vi "Arayuz_v4.vi"() -> ()   [LabVIEW 2014]
uses:
  CustomControls/Program_States.ctl
  <vilib>/Platform/TimedLoop/XDataNode/timing_clust.ctl
  <vilib>/Platform/TimedLoop/XDataNode/nitl_modes.ctl
  <vilib>/Platform/TimedLoop/XDataNode/wakeup.ctl
  CustomControls/TSE_Status.ctl
  SharedVariables/TSE_Variables.vi
  <vilib>/platform/TimedLoop/XDataNode/XDataNode.xnode
  <vilib>/Platform/TimedLoop/XDataNode/XDNodeRunTimeDep.lvlib
panel:
  in  "?":string="GKÇ KALİBRASYON YAZILIMI"
  in  "Sertifika Kaydet":bool=TRUE
  in  "DURDUR":bool
  out "Ring":T1=enum."Durdur"
  in  "Main Tab Control":enum32{"GKÇ 1", "GKÇ 2", "GKÇ 3"}(tab)
  in  "GKÇ-1 Tab Control":T2(tab)
  out "GKÇ-1 Frekans Sonuç Tablosu":string[][](table)
  out "GKÇ-1 Gerilim Sonuç Tablosu":string[][](table)
  out "GKÇ-1 Akım Sonuç Tablosu":string[][](table)
  out "GKÇ-1 Aktif Güç Sonuç Tablosu":string[][](table)
  out "GKÇ-1 Reaktif Güç Sonuç Tablosu":string[][](table)
  out "GKÇ-1 Harmonik Akım Sonuç Tablosu":string[][](table)
  out "GKÇ-1 Harmonik Gerilim Sonuç Tablosu":string[][](table)
  out "GKÇ-1 Flicker Sonuç Tablosu":string[][](table)
  out "Flicker Sonuç":bool caption="Flicker"
  out "Harmonik G. Sonuç":bool caption="Harmonik Gerilim"
  out "Harmonik A. Sonuç":bool caption="Harmonik Akım"
  out "Reaktif G. Sonuç":bool caption="Reaktif Güç"
  out "Aktif G. Sonuç":bool caption="Aktif Güç"
  out "Akım Sonuç":bool caption="AC Akım"
  out "Gerilim Sonuç":bool caption="AC Gerilim"
  out "Mesaj":string="Program Durduruldu !"
  out "Frekans Sonuç":bool caption="Frekans"
  in  "Dosya Adı":path
  in  "BAŞLAT":bool
  # "Uygulanan Değer"
  # "Hata_Fider 1"
  # "Hata_Fider 2"
  # "Sonuç"
  # "Uygulanan Değer"
  # "Hata_Fider 1"
  # "Hata_Fider 2"
  # "Sonuç"
  # "Uygulanan Değer"
  # "Hata_Fider 1"
  # "Hata_Fider 2"
  # "Sonuç"
  # "Uygulanan Değer"
  # "Hata_Fider 1"
  # "Hata_Fider 2"
  # "Sonuç"
  # "Uygulanan Değer"
  # "Hata_Fider 1"
  # "Hata_Fider 2"
  # "Sonuç"
  # "Uygulanan Değer"
  # "Hata_Fider 1"
  # "Hata_Fider 2"
  # "Sonuç"
  # "Uygulanan Değer"
  # "Hata_Fider 1"
  # "Hata_Fider 2"
  # "Sonuç"
  # "Uygulanan Değer"
  # "Hata_Fider 1"
  # "Hata_Fider 2"
  # "Sonuç"
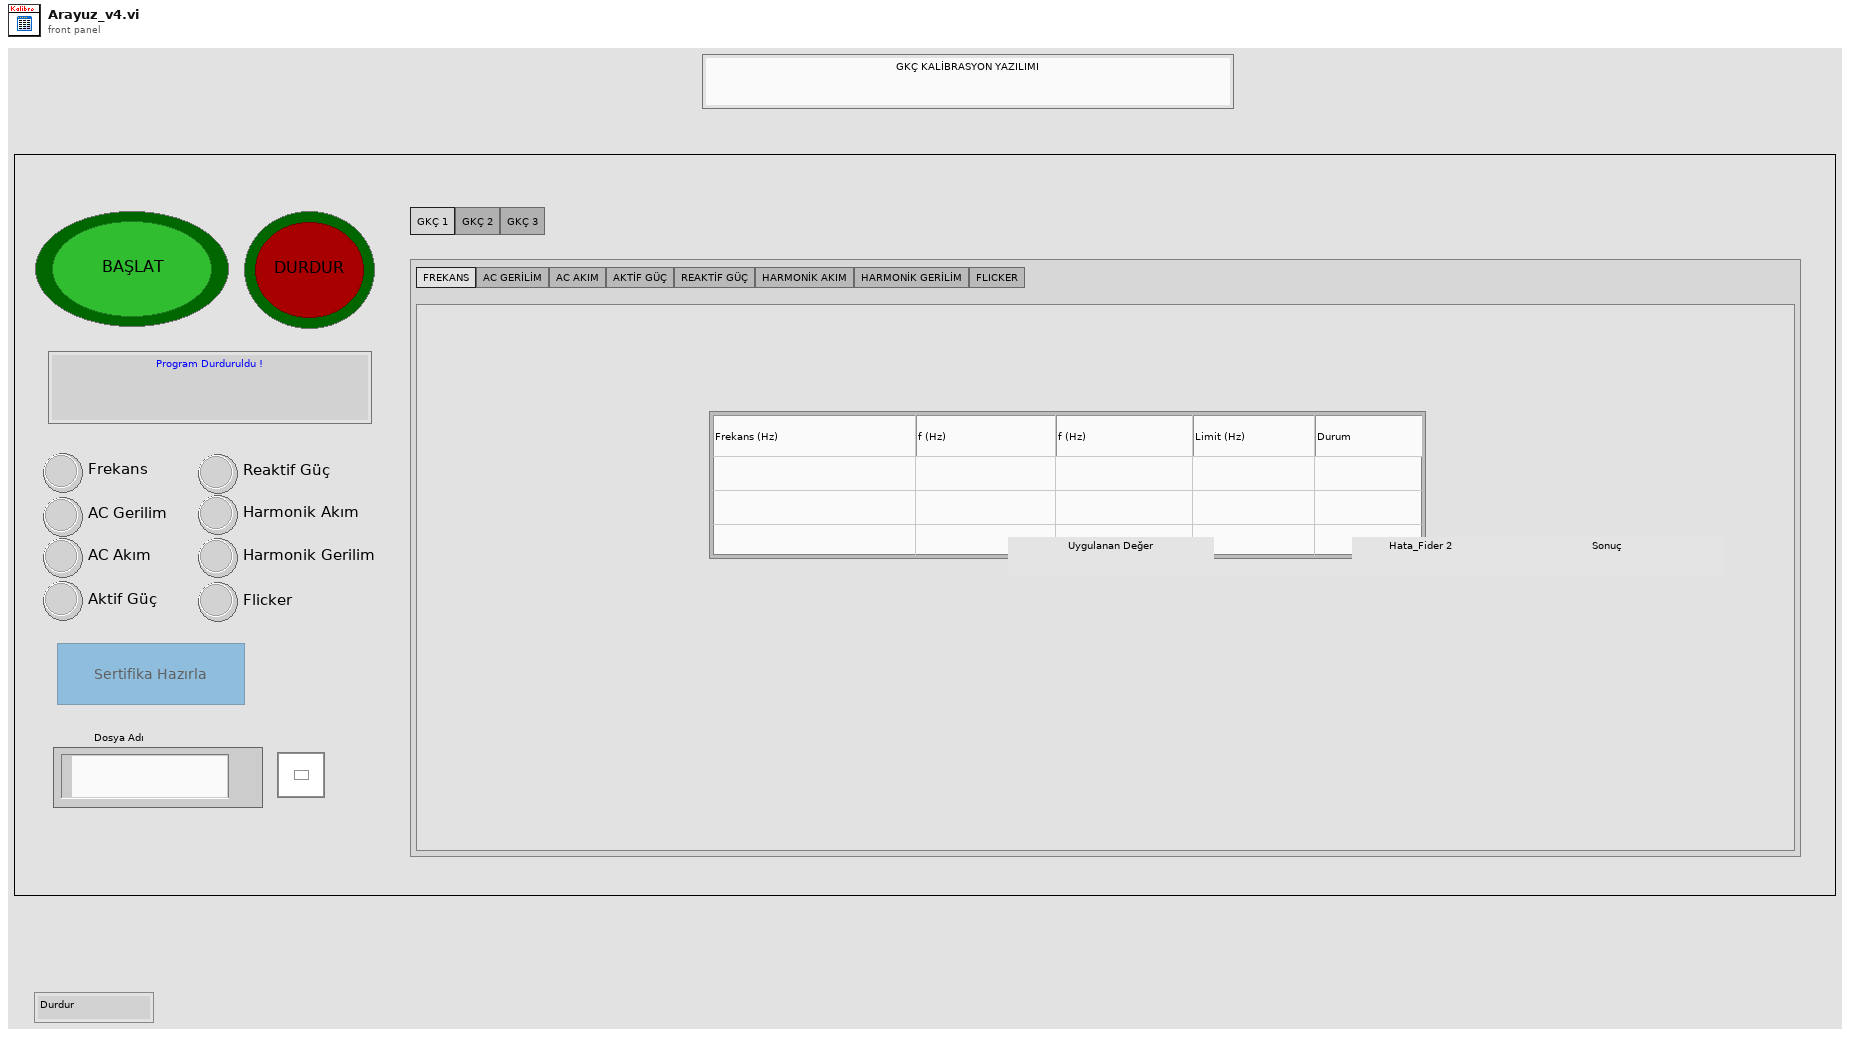
[diagram p1: front panel]
types:
  T1 = typedef "Program_States.ctl" = enum16{"Ön Yükleme", "TSE Baslat", "Kalibratöre Baglan", "Kalibratörü Baslat", "Ön Yükleme Tamam", "Frekans Testi", "Gerilim Testi", "Akim Testi", "Aktif Guc Testi", "Reaktif Guc Testi", "AC Akim Harmonik Testi", "AC Gerilim Harmonik Testi", "Flicker Testi", "Rapor Cikarma", "Yeniden Başlat", "Bekleme", "Durdur"}
  T2 = enum32{"FREKANS", "AC GERİLİM", "AC AKIM", "AKTİF GÜÇ", "REAKTİF GÜÇ", "HARMONİK AKIM", "HARMONİK GERİLİM", "FLICKER"}
  T3 = cluster{"Test A. Süresi":i32, "Iterasyon Sayisi":i32}
  T4 = typedef "TSE_Status.ctl" = cluster{"Return Code":i32, "Message":string, "error in (no error)":errorcluster, "Program State":T1, "Test A. Suresi":u32}
  T5 = typedef "XDNodeRunTimeDep.lvlib/timing_clust.ctl" = cluster{"Expected End [f-1]":u64, "Actual End [f-1]":u64, "Finished Late? [f-1]":bool, "Expected End [i-1]":u64, "Actual End [i-1]":u64, "Finished Late? [i-1]":bool, "Expected Start [i]":u64, "Actual Start [i]":u64, "Expected Start [f]":u64, "Actual Start [f]":u64, "Source Name":string, "Structure Name":string, "Period":i64, "Deadline":i64, "Offset":i64, "Start":i64, "Priority":i32, "Timeout":i32, "Mode":T6, "Wakeup Reason":T7, "Error":errorcluster, "Source Type":string, "Secondary Source Type":string, "Global End Time":u64, "Global Start Time":u64, "Frame Duration":u64, "Iteration Duration":u64, "Assigned CPU":i32, "I/O Scan Engine Mode":u32}
  T6 = typedef "XDNodeRunTimeDep.lvlib/nitl_modes.ctl" = enum32{"No Change", "Process missed periods, maintain original phase", "Discard missed periods, maintain original phase", "Process missed periods, ignore original phase", "Discard missed periods, ignore original phase"}
  T7 = typedef "XDNodeRunTimeDep.lvlib/wakeup.ctl" = enum32{"Normal", "Aborted", "Asynchronous wakeup", "Timing source error", "Timed loop error", "Timeout"}
  T8 = enum8{"Enabled", "Disabled", "Disabled and Grayed Out"}
  T9 = enum32{"invalid app kind", "Development System", "Run Time System", "Student Edition", "Embedded LabVIEW", "Evaluation", "Custom"}
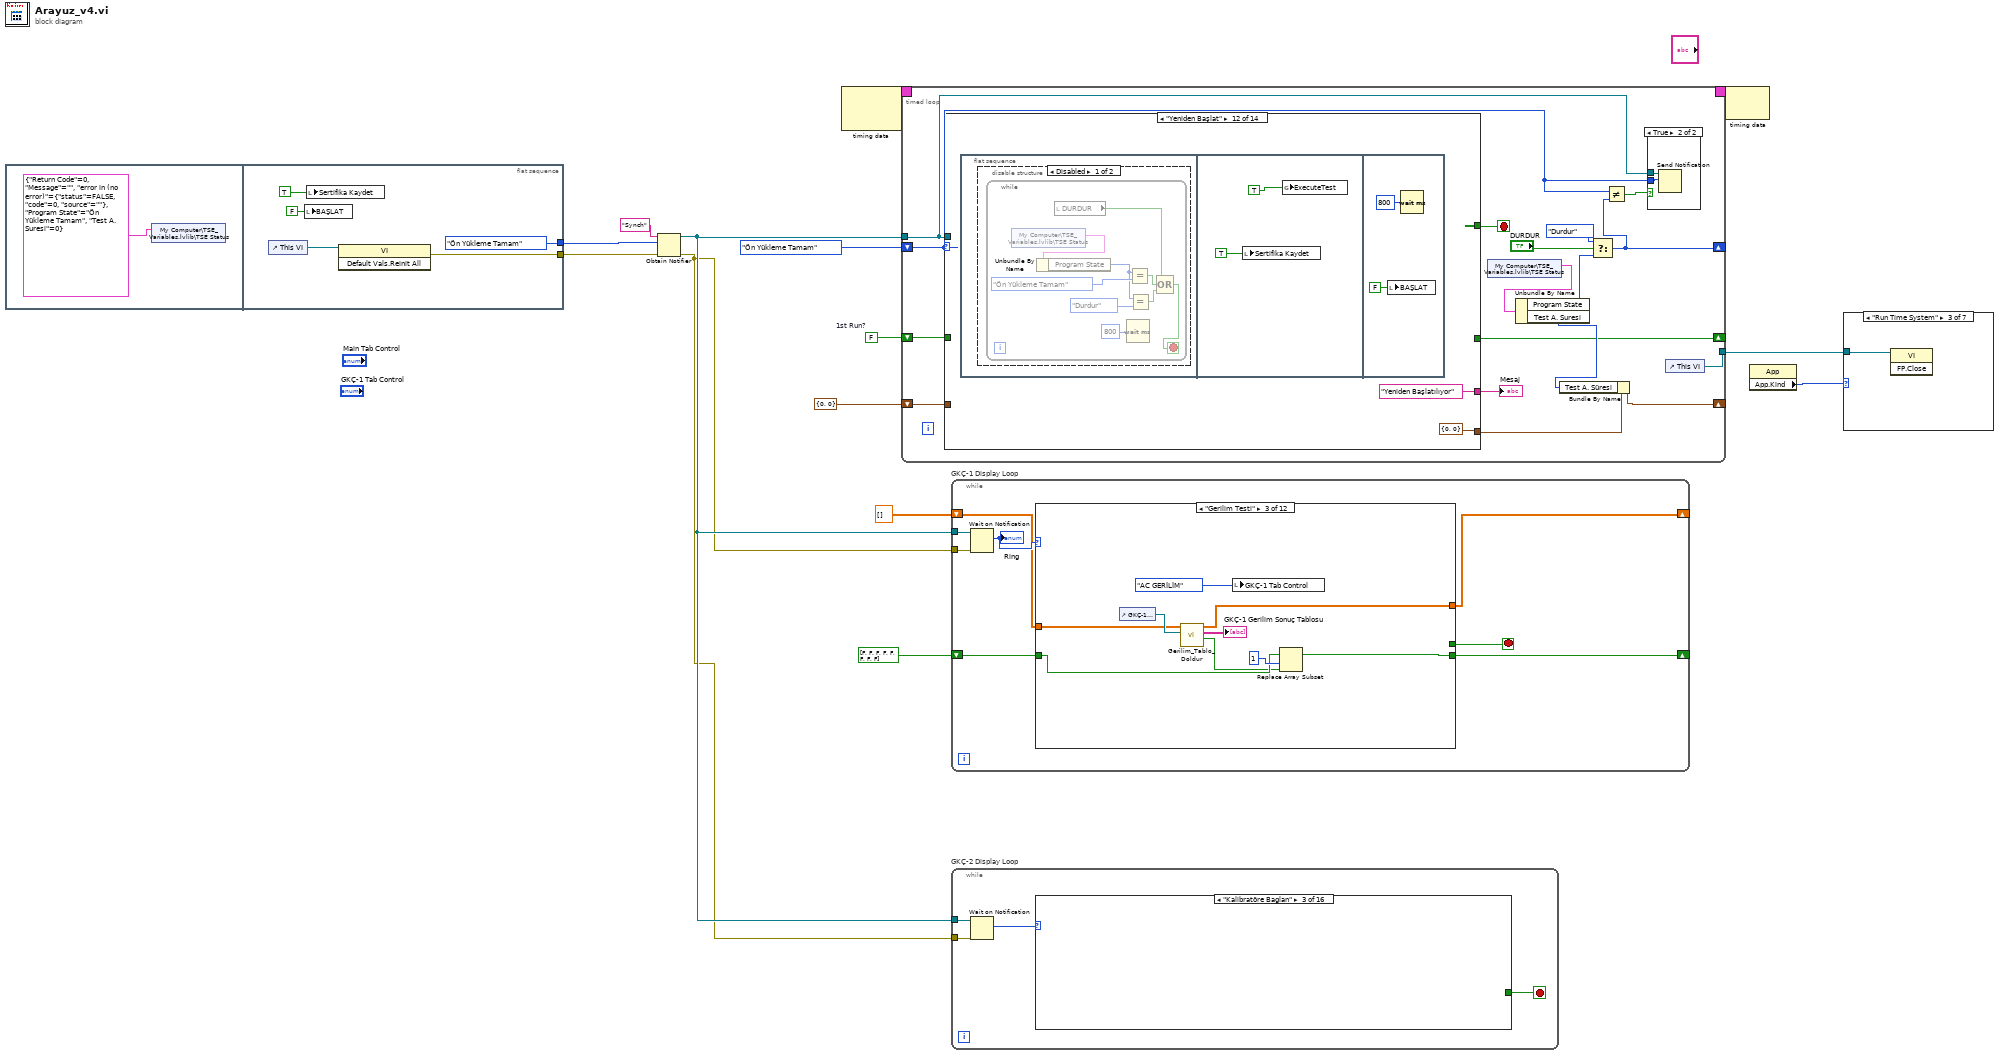
[diagram p0: block diagram]
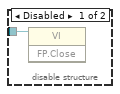
[diagram p4: hidden frame]
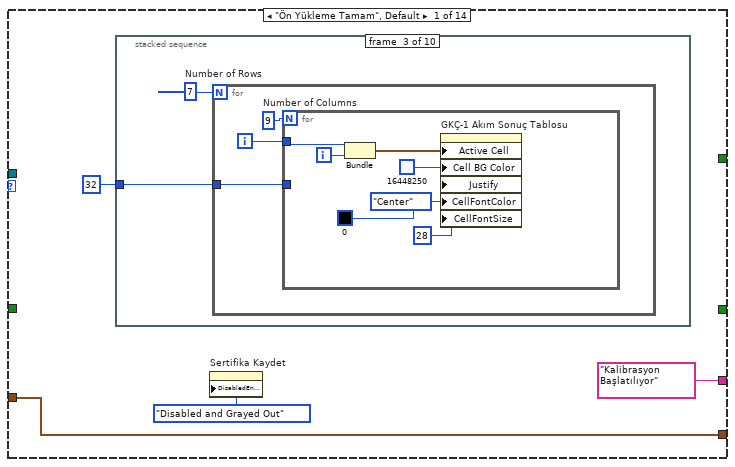
[diagram p10: hidden frame]
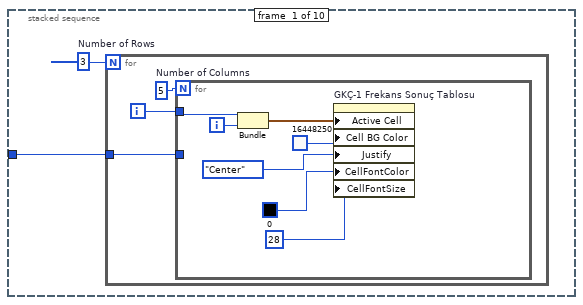
[diagram p11: hidden frame]
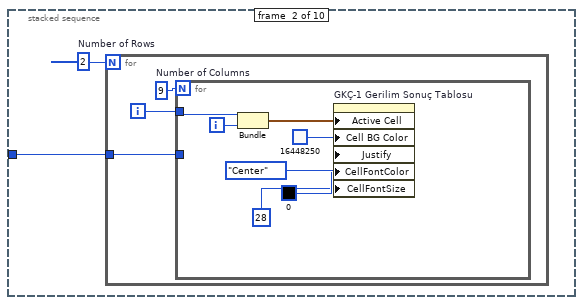
[diagram p12: hidden frame]
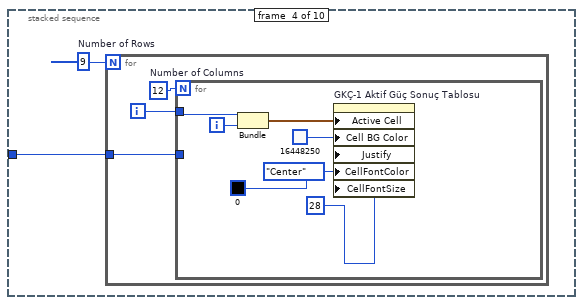
[diagram p13: hidden frame]
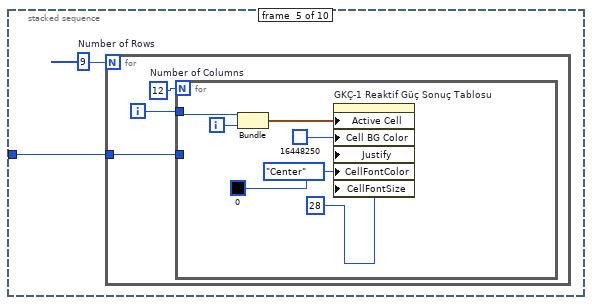
[diagram p14: hidden frame]
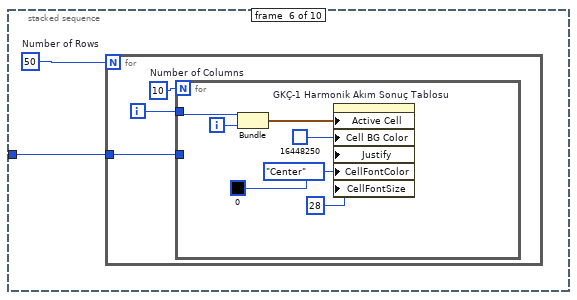
[diagram p15: hidden frame]
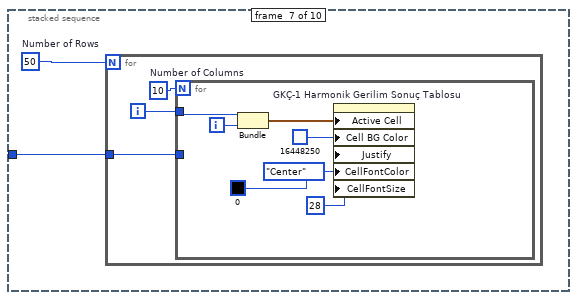
[diagram p16: hidden frame]
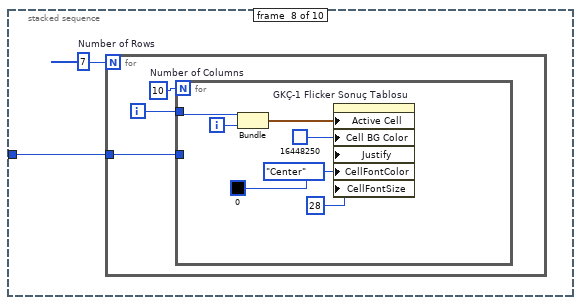
[diagram p17: hidden frame]
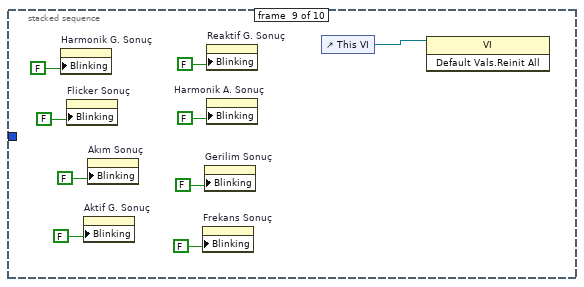
[diagram p18: hidden frame]
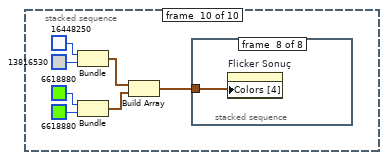
[diagram p19: hidden frame]
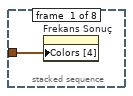
[diagram p20: hidden frame]
diagram:
  w2 = FALSE  # 1st Run?
  n1 = flat-sequence {
    tunnel: [Program_States."Ön Yükleme Tamam" ("Ring")] -> w13
    tunnel: [w18] -> w6
    frame #0 {
      n2 = shared-variable "My Computer\\TSE_Variables.lvlib\\TSE Status"(T4 {"Return Code"=0, "Message"="", "error in (no error)"={"status"=FALSE, "code"=0, "source"=""}, "Program State"=enum."Ön Yükleme Tamam", "Test A. Suresi"=0} ("TSE Status")) -> ()  [unwired: 1 in, 1 out]
    }
    frame #1 {
      n3 = control-ref of="This VI"() -> (w19:refnum<vi>)
      n4 = local write "BAŞLAT"(FALSE ("BAŞLAT")) -> ()
      n5 = local write "Sertifika Kaydet"(TRUE ("Sertifika Kaydet")) -> ()
      n6 = invoke class="VI" method="Default Vals.Reinit All"(reference=w19) -> (error out=w18:errorcluster)  [unwired: 2 in, 2 out]
    }
  }
  n7 = Obtain Notifier(name (unnamed)="Synch", notification data type=w13, error in (no error)=w6) -> (notifier out=w11:refnum<notifier>, error out=w10:errorcluster)  [unwired: 1 in, 1 out]
  n8 = node-c288() -> (w8:T5)  [unwired: 2 in]
  n9 = timed-loop {
    tunnel: w11 -> [w26]
    shift-right: [w27] -> _
    shift-left: Program_States."Ön Yükleme Tamam" ("Ring") -> [w24]
    shift-right: [w33] -> _
    shift-left: T3 {"Test A. Süresi"=0, "Iterasyon Sayisi"=0} -> [w37]
    timing: w8 -> [_]
    timing-out: [_] -> w7
    tunnel: [w28] -> w5
    shift-right: [w22] -> _
    shift-left: w2 -> [w23]
    stop <- w31 stop-if-true
    n10 = case shown="\"Yeniden Başlat\"" w24 {
      selector: w24 -> [_ _ _ _ _ _ _ _ _ _ _ _ w315 w326]
      tunnel: w37 -> [w43 _ w173 w184 w199 w214 w230 w243 w258 w273 _ _ _ w329]
      tunnel: [w43 _ w170 w181 w196 w211 w227 w240 w255 w270 _ T3 {"Test A. Süresi"=0, "Iterasyon Sayisi"=0} _ w328] -> w36
      tunnel: [_ _ FALSE FALSE FALSE FALSE FALSE FALSE FALSE FALSE _ _ TRUE _] -> w31
      tunnel: ["Kalibrasyon Başlatılıyor" "" "Frekans Ölçümü\nDevam Ediyor" w186 w201 w216 "Reaktif Güç Ölçümü\nDevam Ediyor" w245 w260 w275 "Ölçümler Tamamlandı" "Yeniden Başlatılıyor" "Program Durduruldu !" "Bekleniyor..."] -> w30
      tunnel: w26 -> [_ _ _ _ _ _ _ _ _ _ w285 _ w316 w325]
      tunnel: w23 -> [_ _ w167 w179 w194 w209 w224 w238 w253 w268 _ _ _ _]
      tunnel: [_ TRUE _ w178 w193 w208 w223 w237 w252 w267 _ _ _ _] -> w22
      frame "Ön Yükleme Tamam", Default {
        n11 = stacked-sequence {
          tunnel: u32 32 ("Active Cell:Cell Size:Height") -> [w44 w56 w68 w80 w92 w104 w116 w128 _ _]
          frame #0 {
            w45 = 3  # Number of Rows
            n12 = for {
              N: w45 -> [_]
              tunnel: w44 -> [w47]
              i -> [w48]
              w46 = 5  # Number of Columns
              n13 = for {
                N: w46 -> [_]
                tunnel: w48 -> [w55]
                tunnel: w47 -> [_]
                i -> [w52]
                n14 = Bundle(w55, w52) -> (w54:cluster{i32, i32})  [unwired: 1 in]
                n15 = property on="GKÇ-1 Frekans Sonuç Tablosu" class="Tbl (strict)"("Active Cell"=w54, "Cell BG Color"=u32 16448250, "Justify"=enum16{"Left", "Center", "Right"}."Center" ("Active Cell:Cell Justification"), "CellFontColor"=u32 0, "CellFontSize"=u32 28 ("Active Cell:Cell Font:Size")) -> ()  [unwired: 2 in, 2 out]
              }
            }
          }
          frame #1 {
            w57 = 2  # Number of Rows
            n16 = for {
              N: w57 -> [_]
              tunnel: w56 -> [w59]
              i -> [w60]
              w58 = 9  # Number of Columns
              n17 = for {
                N: w58 -> [_]
                tunnel: w60 -> [w67]
                tunnel: w59 -> [_]
                i -> [w64]
                n18 = Bundle(w67, w64) -> (w66:cluster{i32, i32})  [unwired: 1 in]
                n19 = property on="GKÇ-1 Gerilim Sonuç Tablosu" class="Tbl (strict)"("Active Cell"=w66, "Cell BG Color"=u32 16448250, "Justify"=enum16{"Left", "Center", "Right"}."Center" ("Active Cell:Cell Justification"), "CellFontColor"=u32 0, "CellFontSize"=u32 28 ("Active Cell:Cell Font:Size")) -> ()  [unwired: 2 in, 2 out]
              }
            }
          }
          frame #2 {
            w69 = 7  # Number of Rows
            n20 = for {
              N: w69 -> [_]
              tunnel: w68 -> [w71]
              i -> [w72]
              w70 = 9  # Number of Columns
              n21 = for {
                N: w70 -> [_]
                tunnel: w72 -> [w79]
                tunnel: w71 -> [_]
                i -> [w76]
                n22 = Bundle(w79, w76) -> (w78:cluster{i32, i32})  [unwired: 1 in]
                n23 = property on="GKÇ-1 Akım Sonuç Tablosu" class="Tbl (strict)"("Active Cell"=w78, "Cell BG Color"=u32 16448250, "Justify"=enum16{"Left", "Center", "Right"}."Center" ("Active Cell:Cell Justification"), "CellFontColor"=u32 0, "CellFontSize"=u32 28 ("Active Cell:Cell Font:Size")) -> ()  [unwired: 2 in, 2 out]
              }
            }
          }
          frame #3 {
            w81 = 9  # Number of Rows
            n24 = for {
              N: w81 -> [_]
              tunnel: w80 -> [w83]
              i -> [w84]
              w82 = 12  # Number of Columns
              n25 = for {
                N: w82 -> [_]
                tunnel: w84 -> [w91]
                tunnel: w83 -> [_]
                i -> [w88]
                n26 = Bundle(w91, w88) -> (w90:cluster{i32, i32})  [unwired: 1 in]
                n27 = property on="GKÇ-1 Aktif Güç Sonuç Tablosu" class="Tbl (strict)"("Active Cell"=w90, "Cell BG Color"=u32 16448250, "Justify"=enum16{"Left", "Center", "Right"}."Center" ("Active Cell:Cell Justification"), "CellFontColor"=u32 0, "CellFontSize"=u32 28 ("Active Cell:Cell Font:Size")) -> ()  [unwired: 2 in, 2 out]
              }
            }
          }
          frame #4 {
            w93 = 9  # Number of Rows
            n28 = for {
              N: w93 -> [_]
              tunnel: w92 -> [w95]
              i -> [w96]
              w94 = 12  # Number of Columns
              n29 = for {
                N: w94 -> [_]
                tunnel: w96 -> [w103]
                tunnel: w95 -> [_]
                i -> [w100]
                n30 = Bundle(w103, w100) -> (w102:cluster{i32, i32})  [unwired: 1 in]
                n31 = property on="GKÇ-1 Reaktif Güç Sonuç Tablosu" class="Tbl (strict)"("Active Cell"=w102, "Cell BG Color"=u32 16448250, "Justify"=enum16{"Left", "Center", "Right"}."Center" ("Active Cell:Cell Justification"), "CellFontColor"=u32 0, "CellFontSize"=u32 28 ("Active Cell:Cell Font:Size")) -> ()  [unwired: 2 in, 2 out]
              }
            }
          }
          frame #5 {
            w105 = 50  # Number of Rows
            n32 = for {
              N: w105 -> [_]
              tunnel: w104 -> [w107]
              i -> [w108]
              w106 = 10  # Number of Columns
              n33 = for {
                N: w106 -> [_]
                tunnel: w108 -> [w115]
                tunnel: w107 -> [_]
                i -> [w112]
                n34 = Bundle(w115, w112) -> (w114:cluster{i32, i32})  [unwired: 1 in]
                n35 = property on="GKÇ-1 Harmonik Akım Sonuç Tablosu" class="Tbl (strict)"("Active Cell"=w114, "Cell BG Color"=u32 16448250, "Justify"=enum16{"Left", "Center", "Right"}."Center" ("Active Cell:Cell Justification"), "CellFontColor"=u32 0, "CellFontSize"=u32 28 ("Active Cell:Cell Font:Size")) -> ()  [unwired: 2 in, 2 out]
              }
            }
          }
          frame #6 {
            w117 = 50  # Number of Rows
            n36 = for {
              N: w117 -> [_]
              tunnel: w116 -> [w119]
              i -> [w120]
              w118 = 10  # Number of Columns
              n37 = for {
                N: w118 -> [_]
                tunnel: w120 -> [w127]
                tunnel: w119 -> [_]
                i -> [w124]
                n38 = Bundle(w127, w124) -> (w126:cluster{i32, i32})  [unwired: 1 in]
                n39 = property on="GKÇ-1 Harmonik Gerilim Sonuç Tablosu" class="Tbl (strict)"("Active Cell"=w126, "Cell BG Color"=u32 16448250, "Justify"=enum16{"Left", "Center", "Right"}."Center" ("Active Cell:Cell Justification"), "CellFontColor"=u32 0, "CellFontSize"=u32 28 ("Active Cell:Cell Font:Size")) -> ()  [unwired: 2 in, 2 out]
              }
            }
          }
          frame #7 {
            w129 = 7  # Number of Rows
            n40 = for {
              N: w129 -> [_]
              tunnel: w128 -> [w131]
              i -> [w132]
              w130 = 10  # Number of Columns
              n41 = for {
                N: w130 -> [_]
                tunnel: w132 -> [w139]
                tunnel: w131 -> [_]
                i -> [w136]
                n42 = Bundle(w139, w136) -> (w138:cluster{i32, i32})  [unwired: 1 in]
                n43 = property on="GKÇ-1 Flicker Sonuç Tablosu" class="Tbl (strict)"("Active Cell"=w138, "Cell BG Color"=u32 16448250, "Justify"=enum16{"Left", "Center", "Right"}."Center" ("Active Cell:Cell Justification"), "CellFontColor"=u32 0, "CellFontSize"=u32 28 ("Active Cell:Cell Font:Size")) -> ()  [unwired: 2 in, 2 out]
              }
            }
          }
          frame #8 {
            n44 = property on="Harmonik G. Sonuç" class="Bool (strict)"("Blinking"=FALSE) -> ()  [unwired: 2 in, 2 out]
            n45 = property on="Flicker Sonuç" class="Bool (strict)"("Blinking"=FALSE) -> ()  [unwired: 2 in, 2 out]
            n46 = property on="Aktif G. Sonuç" class="Bool (strict)"("Blinking"=FALSE) -> ()  [unwired: 2 in, 2 out]
            n47 = property on="Akım Sonuç" class="Bool (strict)"("Blinking"=FALSE) -> ()  [unwired: 2 in, 2 out]
            n48 = property on="Frekans Sonuç" class="Bool (strict)"("Blinking"=FALSE) -> ()  [unwired: 2 in, 2 out]
            n49 = property on="Gerilim Sonuç" class="Bool (strict)"("Blinking"=FALSE) -> ()  [unwired: 2 in, 2 out]
            n50 = property on="Reaktif G. Sonuç" class="Bool (strict)"("Blinking"=FALSE) -> ()  [unwired: 2 in, 2 out]
            n51 = property on="Harmonik A. Sonuç" class="Bool (strict)"("Blinking"=FALSE) -> ()  [unwired: 2 in, 2 out]
            n52 = control-ref of="This VI"() -> (w148:refnum<vi>)
            n53 = invoke class="VI" method="Default Vals.Reinit All"(reference=w148) -> ()  [unwired: 2 in, 3 out]
          }
          frame #9 {
            n54 = Bundle(u32 16448250, u32 13816530) -> (w152:cluster{u32, u32})  [unwired: 1 in]
            n55 = Bundle(u32 6618880, u32 6618880) -> (w149:cluster{u32, u32})  [unwired: 1 in]
            n56 = Build Array(w152, w149) -> (w155:cluster{u32, u32}[])
            n57 = stacked-sequence {
              tunnel: w155 -> [w156 w157 w158 w159 w160 w161 w162 w163]
              frame #0 {
                n58 = property on="Frekans Sonuç" class="Bool (strict)"("Colors [4]"=w156) -> ()  [unwired: 2 in, 2 out]
              }
              frame #1 {
                n59 = property on="Gerilim Sonuç" class="Bool (strict)"("Colors [4]"=w157) -> ()  [unwired: 2 in, 2 out]
              }
              frame #2 {
                n60 = property on="Akım Sonuç" class="Bool (strict)"("Colors [4]"=w158) -> ()  [unwired: 2 in, 2 out]
              }
              frame #3 {
                n61 = property on="Aktif G. Sonuç" class="Bool (strict)"("Colors [4]"=w159) -> ()  [unwired: 2 in, 2 out]
              }
              frame #4 {
                n62 = property on="Reaktif G. Sonuç" class="Bool (strict)"("Colors [4]"=w160) -> ()  [unwired: 2 in, 2 out]
              }
              frame #5 {
                n63 = property on="Harmonik A. Sonuç" class="Bool (strict)"("Colors [4]"=w161) -> ()  [unwired: 2 in, 2 out]
              }
              frame #6 {
                n64 = property on="Harmonik G. Sonuç" class="Bool (strict)"("Colors [4]"=w162) -> ()  [unwired: 2 in, 2 out]
              }
              frame #7 {
                n65 = property on="Flicker Sonuç" class="Bool (strict)"("Colors [4]"=w163) -> ()  [unwired: 2 in, 2 out]
              }
            }
          }
        }
        n66 = property on="Sertifika Kaydet" class="Bool (strict)"("DisabledEnum"=T8."Disabled and Grayed Out" ("Disabled")) -> ()  [unwired: 2 in, 2 out]
      }
      frame "Ön Yükleme" {
      }
      frame "Frekans Testi" {
        n67 = Unbundle By Name(w173) -> ("Iterasyon Sayisi"=w172:i32)
        n68 = property on="Frekans Sonuç" class="Bool (strict)"("Blinking"=TRUE) -> ()  [unwired: 2 in, 2 out]
        n69 = Increment(x=w172) -> (x+1=w171:i32)
        n70 = case shown="True" w167 {
          selector: w167 -> [w174 _]
          tunnel: [w174 FALSE] -> _
          frame False {
          }
          frame True {
            n71 = local write "GKÇ-1 Tab Control"(T2."FREKANS" ("GKÇ-1 Tab Control")) -> ()
          }
        }
        n72 = Bundle By Name(cluster=w173, "Iterasyon Sayisi"=w171) -> (w170:T3)
      }
      frame "Gerilim Testi" {
        n73 = Unbundle By Name(w184) -> ("Iterasyon Sayisi"=w183:i32)
        n74 = property on="Gerilim Sonuç" class="Bool (strict)"("Blinking"=TRUE) -> ()  [unwired: 2 in, 2 out]
        n75 = Increment(x=w183) -> (x+1=w182:i32)
        n76 = case shown="True" w179 {
          selector: w179 -> [w187 _]
          tunnel: [w187 FALSE] -> w178
          frame False {
          }
          frame True {
            n77 = property on="Frekans Sonuç" class="Bool (strict)"("Blinking"=FALSE) -> ()  [unwired: 2 in, 2 out]
            n78 = call "Sonuç_Led_Rengi.vi"() -> ("Array"=w188:cluster{u32, u32}[])
            n79 = property on="Frekans Sonuç" class="Bool (strict)"("Colors [4]"=w188) -> ()  [unwired: 2 in, 2 out]
            n80 = local write "GKÇ-1 Tab Control"(T2."AC GERİLİM" ("GKÇ-1 Tab Control")) -> ()
          }
        }
        n81 = Bundle By Name(cluster=w184, "Iterasyon Sayisi"=w182) -> (w181:T3)
        n82 = Concatenate Strings("Gerilim Ölçümü\nDevam Ediyor ") -> (w186:string)
      }
      frame "Akim Testi" {
        n83 = Unbundle By Name(w199) -> ("Iterasyon Sayisi"=w198:i32)
        n84 = property on="Akım Sonuç" class="Bool (strict)"("Blinking"=TRUE) -> ()  [unwired: 2 in, 2 out]
        n85 = Increment(x=w198) -> (x+1=w197:i32)
        n86 = case shown="True" w194 {
          selector: w194 -> [w202 _]
          tunnel: [w202 FALSE] -> w193
          frame False {
          }
          frame True {
            n87 = property on="Gerilim Sonuç" class="Bool (strict)"("Blinking"=FALSE) -> ()  [unwired: 2 in, 2 out]
            n88 = call "Sonuç_Led_Rengi.vi"() -> ("Array"=w203:cluster{u32, u32}[])
            n89 = property on="Gerilim Sonuç" class="Bool (strict)"("Colors [4]"=w203) -> ()  [unwired: 2 in, 2 out]
            n90 = local write "GKÇ-1 Tab Control"(T2."AC AKIM" ("GKÇ-1 Tab Control")) -> ()
          }
        }
        n91 = Bundle By Name(cluster=w199, "Iterasyon Sayisi"=w197) -> (w196:T3)
        n92 = Concatenate Strings("Akım Ölçümü\nDevam Ediyor") -> (w201:string)
      }
      frame "Aktif Guc Testi" {
        n93 = Unbundle By Name(w214) -> ("Iterasyon Sayisi"=w213:i32)
        n94 = property on="Aktif G. Sonuç" class="Bool (strict)"("Blinking"=TRUE) -> ()  [unwired: 2 in, 2 out]
        n95 = Increment(x=w213) -> (x+1=w212:i32)
        n96 = case shown="True" w209 {
          selector: w209 -> [w217 _]
          tunnel: [w217 FALSE] -> w208
          frame False {
          }
          frame True {
            n97 = call "Sonuç_Led_Rengi.vi"() -> ("Array"=w218:cluster{u32, u32}[])
            n98 = property on="Akım Sonuç" class="Bool (strict)"("Blinking"=FALSE) -> ()  [unwired: 2 in, 2 out]
            n99 = property on="Akım Sonuç" class="Bool (strict)"("Colors [4]"=w218) -> ()  [unwired: 2 in, 2 out]
            n100 = local write "GKÇ-1 Tab Control"(T2."AKTİF GÜÇ" ("GKÇ-1 Tab Control")) -> ()
          }
        }
        n101 = Bundle By Name(cluster=w214, "Iterasyon Sayisi"=w212) -> (w211:T3)
        n102 = Concatenate Strings("Aktif Güç Ölçümü\nDevam Ediyor") -> (w216:string)
      }
      frame "Reaktif Guc Testi" {
        n103 = Unbundle By Name(w230) -> ("Iterasyon Sayisi"=w229:i32)
        n104 = property on="Reaktif G. Sonuç" class="Bool (strict)"("Blinking"=TRUE) -> ()  [unwired: 2 in, 2 out]
        n105 = Increment(x=w229) -> (x+1=w228:i32)
        n106 = case shown="True" w224 {
          selector: w224 -> [w231 _]
          tunnel: [w231 FALSE] -> w223
          frame False {
          }
          frame True {
            n107 = property on="Aktif G. Sonuç" class="Bool (strict)"("Blinking"=FALSE) -> ()  [unwired: 2 in, 2 out]
            n108 = call "Sonuç_Led_Rengi.vi"() -> ("Array"=w232:cluster{u32, u32}[])
            n109 = property on="Aktif G. Sonuç" class="Bool (strict)"("Colors [4]"=w232) -> ()  [unwired: 2 in, 2 out]
            n110 = local write "GKÇ-1 Tab Control"(T2."REAKTİF GÜÇ" ("GKÇ-1 Tab Control")) -> ()
          }
        }
        n111 = Bundle By Name(cluster=w230, "Iterasyon Sayisi"=w228) -> (w227:T3)
      }
      frame "AC Akim Harmonik Testi" {
        n112 = Unbundle By Name(w243) -> ("Iterasyon Sayisi"=w242:i32)
        n113 = property on="Harmonik A. Sonuç" class="Bool (strict)"("Blinking"=TRUE) -> ()  [unwired: 2 in, 2 out]
        n114 = Increment(x=w242) -> (x+1=w241:i32)
        n115 = case shown="True" w238 {
          selector: w238 -> [w246 _]
          tunnel: [w246 FALSE] -> w237
          frame False {
          }
          frame True {
            n116 = call "Sonuç_Led_Rengi.vi"() -> ("Array"=w247:cluster{u32, u32}[])
            n117 = property on="Reaktif G. Sonuç" class="Bool (strict)"("Blinking"=FALSE) -> ()  [unwired: 2 in, 2 out]
            n118 = property on="Reaktif G. Sonuç" class="Bool (strict)"("Colors [4]"=w247) -> ()  [unwired: 2 in, 2 out]
            n119 = local write "GKÇ-1 Tab Control"(T2."HARMONİK AKIM" ("GKÇ-1 Tab Control")) -> ()
          }
        }
        n120 = Bundle By Name(cluster=w243, "Iterasyon Sayisi"=w241) -> (w240:T3)
        n121 = Concatenate Strings("Harmonik Akım Ölçümü\nDevam Ediyor") -> (w245:string)
      }
      frame "AC Gerilim Harmonik Testi" {
        n122 = Unbundle By Name(w258) -> ("Iterasyon Sayisi"=w257:i32)
        n123 = property on="Harmonik G. Sonuç" class="Bool (strict)"("Blinking"=TRUE) -> ()  [unwired: 2 in, 2 out]
        n124 = Increment(x=w257) -> (x+1=w256:i32)
        n125 = case shown="True" w253 {
          selector: w253 -> [w261 _]
          tunnel: [w261 FALSE] -> w252
          frame False {
          }
          frame True {
            n126 = property on="Harmonik A. Sonuç" class="Bool (strict)"("Blinking"=FALSE) -> ()  [unwired: 2 in, 2 out]
            n127 = call "Sonuç_Led_Rengi.vi"() -> ("Array"=w262:cluster{u32, u32}[])
            n128 = property on="Harmonik A. Sonuç" class="Bool (strict)"("Colors [4]"=w262) -> ()  [unwired: 2 in, 2 out]
            n129 = local write "GKÇ-1 Tab Control"(T2."HARMONİK GERİLİM" ("GKÇ-1 Tab Control")) -> ()
          }
        }
        n130 = Bundle By Name(cluster=w258, "Iterasyon Sayisi"=w256) -> (w255:T3)
        n131 = Concatenate Strings("Harmonik Gerilim Ölçümü\nDevam Ediyor") -> (w260:string)
      }
      frame "Flicker Testi" {
        n132 = Unbundle By Name(w273) -> ("Iterasyon Sayisi"=w272:i32)
        n133 = property on="Flicker Sonuç" class="Bool (strict)"("Blinking"=TRUE) -> ()  [unwired: 2 in, 2 out]
        n134 = Increment(x=w272) -> (x+1=w271:i32)
        n135 = case shown="True" w268 {
          selector: w268 -> [w276 _]
          tunnel: [w276 FALSE] -> w267
          frame False {
          }
          frame True {
            n136 = call "Sonuç_Led_Rengi.vi"() -> ("Array"=w277:cluster{u32, u32}[])
            n137 = property on="Harmonik G. Sonuç" class="Bool (strict)"("Blinking"=FALSE) -> ()  [unwired: 2 in, 2 out]
            n138 = property on="Harmonik G. Sonuç" class="Bool (strict)"("Colors [4]"=w277) -> ()  [unwired: 2 in, 2 out]
            n139 = local write "GKÇ-1 Tab Control"(T2."FLICKER" ("GKÇ-1 Tab Control")) -> ()
          }
        }
        n140 = Bundle By Name(cluster=w273, "Iterasyon Sayisi"=w271) -> (w270:T3)
        n141 = Concatenate Strings("Flicker Ölçümü\nDevam Ediyor") -> (w275:string)
      }
      frame "Rapor Cikarma" {
        n142 = Send Notification(notification=Program_States."Rapor Cikarma", notifier=w285) -> ()  [unwired: 1 in, 2 out]
        n143 = Path To String(path="Dosya Adı") -> (string=w287:string)
        n144 = property on="Sertifika Kaydet" class="Bool (strict)"("DisabledEnum"=T8."Enabled" ("Disabled")) -> (error out=w283:errorcluster)  [unwired: 2 in, 1 out]
        n145 = case shown="False" "Sertifika Kaydet" {
          tunnel: w287 -> [w299 _]
          tunnel: w283 -> [w297 _]
          frame False {
            n146 = Bundle By Name(cluster=T4 {"Return Code"=0, "Message"="", "error in (no error)"={"status"=FALSE, "code"=0, "source"=""}, "Program State"=enum."Bekleme", "Test A. Suresi"=0} ("TSE Status"), "Message"=w299, "Return Code"=1) -> (w294:T4)
            n147 = local write "Mesaj"("Rapor Hazırlanıyor " ("Mesaj")) -> ()
            n148 = shared-variable "My Computer\\TSE_Variables.lvlib\\TSE Status"(w294) -> ()  [unwired: 1 in, 1 out]
            n149 = property on="Sertifika Kaydet" class="Bool (strict)"(error in=w297, "DisabledEnum"=T8."Disabled and Grayed Out" ("Disabled")) -> ()  [unwired: 1 in, 2 out]
          }
          frame True {
          }
        }
        n150 = call "Sonuç_Led_Rengi.vi"() -> ("Array"=w281:cluster{u32, u32}[])
        n151 = property on="Flicker Sonuç" class="Bool (strict)"("Blinking"=FALSE) -> ()  [unwired: 2 in, 2 out]
        n152 = property on="Flicker Sonuç" class="Bool (strict)"("Colors [4]"=w281) -> ()  [unwired: 2 in, 2 out]
        n153 = case shown="True" "BAŞLAT" {
          frame False {
          }
          frame True {
            n154 = shared-variable "My Computer\\TSE_Variables.lvlib\\TSE Status"(T4 {"Return Code"=0, "Message"="", "error in (no error)"={"status"=FALSE, "code"=0, "source"=""}, "Program State"=enum."Yeniden Başlat", "Test A. Suresi"=0} ("TSE Status")) -> ()  [unwired: 1 in, 1 out]
          }
        }
      }
      frame "Yeniden Başlat" {
        n155 = flat-sequence {
          frame #0 {
            n156 = disable-structure shown="Disabled" {
              frame Disabled {
                n157 = while {
                  stop <- w306 stop-if-true
                  n158 = shared-variable "My Computer\\TSE_Variables.lvlib\\TSE Status"() -> (w303:T4)  [unwired: 1 in, 1 out]
                  n159 = Unbundle By Name(w303) -> ("Program State"=w302:T1)
                  n160 = local read "DURDUR"() -> (w305:bool)
                  n161 = Wait (ms)(milliseconds to wait=u32 800) -> ()  [unwired: 1 out]
                  n162 = Equal?(x=w302, y=Program_States."Ön Yükleme Tamam") -> (x = y?=w308:bool)
                  n163 = Equal?(x=w302, y=Program_States."Durdur") -> (x = y?=w307:bool)
                  n164 = Compound Arithmetic op=OR(w305, w308, w307) -> (w306:bool)
                }
              }
              frame Enabled {
              }
            }
          }
          frame #1 {
            n165 = local write "Sertifika Kaydet"(TRUE ("Sertifika Kaydet")) -> ()
            n166 = global write "TSE_Variables.vi" "ExecuteTest"(TRUE ("ExecuteTest")) -> ()
          }
          frame #2 {
            n167 = local write "BAŞLAT"(FALSE ("BAŞLAT")) -> ()
            n168 = Wait (ms)(milliseconds to wait=u32 800) -> ()  [unwired: 1 out]
          }
        }
      }
      frame "Durdur" {
        n169 = Send Notification(notification=w315, notifier=w316) -> ()  [unwired: 1 in, 2 out]
        n170 = flat-sequence {
          frame #0 {
            n171 = shared-variable "My Computer\\TSE_Variables.lvlib\\TSE Status"(T4 {"Return Code"=0, "Message"="", "error in (no error)"={"status"=FALSE, "code"=0, "source"=""}, "Program State"=enum."Durdur", "Test A. Suresi"=0} ("TSE Status")) -> ()  [unwired: 1 in, 1 out]
            n172 = global write "TSE_Variables.vi" "StopTSE"(TRUE ("StopTSE")) -> ()
          }
          frame #1 {
            n173 = local write "Mesaj"("TSE Durduruluyor" ("Mesaj")) -> ()
            n174 = Wait (ms)(milliseconds to wait=u32 800) -> ()  [unwired: 1 out]
          }
          frame #2 {
            n175 = while {
              stop <- w323 continue-if-true
              n176 = shared-variable "My Computer\\TSE_Variables.lvlib\\TS_Executing"() -> (w323:bool)  [unwired: 1 in, 1 out]
              n177 = Wait (ms)(milliseconds to wait=u32 800) -> ()  [unwired: 1 out]
            }
          }
        }
      }
      frame "Bekleme" {
        n178 = disable-structure shown="Enabled" {
          disable-tunnel: w326 -> [w335 _]
          disable-tunnel: w325 -> [w334 _]
          frame Disabled {
            n179 = global read "TSE_Variables.vi" "TSE Status"() -> (w331:T4)
            n180 = Unbundle By Name(w331) -> ("Program State"=w332:T1)
            n181 = Not Equal?(x=w335, y=w332) -> (x != y?=w333:bool)
            n182 = case shown="True" w333 {
              tunnel: w334 -> [_ w337]
              tunnel: w332 -> [_ w336]
              frame False {
              }
              frame True {
                n183 = Send Notification(notification=w336, notifier=w337) -> ()  [unwired: 1 in, 2 out]
              }
            }
          }
          frame Enabled {
            n184 = local read "BAŞLAT"() -> (w338:bool)
            n185 = case shown="True" w338 {
              frame False {
              }
              frame True {
                n186 = shared-variable "My Computer\\TSE_Variables.lvlib\\TSE Status"(T4 {"Return Code"=0, "Message"="", "error in (no error)"={"status"=FALSE, "code"=0, "source"=""}, "Program State"=enum."Yeniden Başlat", "Test A. Suresi"=0} ("TSE Status")) -> ()  [unwired: 1 in, 1 out]
              }
            }
          }
        }
        n187 = Bundle By Name(cluster=w329, "Iterasyon Sayisi"=0) -> (w328:T3)
      }
    }
    "Mesaj" <- w30
    n188 = shared-variable "My Computer\\TSE_Variables.lvlib\\TSE Status"() -> (w21:T4)  [unwired: 1 in, 1 out]
    n189 = Unbundle By Name(w21) -> ("Program State"=w34:T1, "Test A. Suresi"=w32:u32)
    n190 = Bundle By Name(cluster=w36, "Test A. Süresi"=w32) -> (w33:T3)
    n191 = Select(t=Program_States."Durdur" ("Ring"), s="DURDUR", f=w34) -> (s? t:f=w27:T1)
    n192 = Not Equal?(x=w24, y=w27) -> (x != y?=w25:bool)
    n193 = case shown="True" w25 {
      tunnel: w26 -> [_ w39]
      tunnel: w24 -> [_ w38]
      frame False {
      }
      frame True {
        n194 = Send Notification(notification=w38, notifier=w39) -> ()  [unwired: 1 in, 2 out]
      }
    }
    n195 = control-ref of="This VI"() -> (w28:refnum<vi>)
  }
  n196 = while "GKÇ-1 Display Loop" {
    tunnel: w11 -> [w349]
    tunnel: w10 -> [w348]
    shift-right: [w345] -> _
    shift-left: dbl[][] [] ("appended array Out") -> [w344]
    shift-right: [w342] -> _
    shift-left: bool[] [FALSE, FALSE, FALSE, FALSE, FALSE, FALSE, FALSE, FALSE] -> [w343]
    stop <- w346 stop-if-true
    n197 = Wait on Notification(notifier=w349, error in (no error)=w348) -> (notification=w347:T1)  [unwired: 2 in, 3 out]
    "Ring" <- w347
    n198 = case shown="\"Gerilim Testi\"" w347 {
      tunnel: [_ _ _ _ _ _ _ _ _ _ TRUE _] -> w346
      tunnel: w344 -> [w351 w357 w367 w376 w384 w393 _ _ w418 _ _ _]
      tunnel: [w351 w356 w366 w375 w383 w392 dbl[][] [] ("appended array Out") dbl[][] [] ("appended array Out") w417 dbl[][] [] ("appended array Out") dbl[][] [] ("appended array Out") dbl[][] [] ("appended array Out")] -> w345
      tunnel: [w350 w352 w361 w370 w379 w388 w397 w405 w413 w422 w424 w427] -> w342
      tunnel: w343 -> [w350 w354 w363 w372 w381 w390 w400 w407 w415 w422 w424 w427]
      frame "Bekleme", Default {
      }
      frame "Frekans Testi" {
        n199 = local write "GKÇ-1 Tab Control"(T2."FREKANS" ("GKÇ-1 Tab Control")) -> ()
        n200 = control-ref of="GKÇ-1 Frekans Sonuç Tablosu"() -> (w358:refnum<vi>)
        n201 = call "Frekans_Tablo_Doldur.vi"("Table Reference in"=w358, "appended array in"=w357) -> ("Test Result"=w353:bool, "Table Values"=→"GKÇ-1 Frekans Sonuç Tablosu":string[][], "appended array Out"=w356:dbl[][])  [unwired: 7 in]
        n202 = Replace Array Subset(array=w354, new element=w353, index=0) -> (w352:bool[])
      }
      frame "Gerilim Testi" {
        n203 = control-ref of="GKÇ-1 Gerilim Sonuç Tablosu"() -> (w368:refnum<vi>)
        n204 = call "Gerilim_Tablo_Doldur.vi"("Table Reference in"=w368, "appended array in"=w367) -> ("Test Result"=w362:bool, "Table Values"=→"GKÇ-1 Gerilim Sonuç Tablosu":string[][], "appended array Out"=w366:dbl[][])  [unwired: 7 in]
        n205 = local write "GKÇ-1 Tab Control"(T2."AC GERİLİM" ("GKÇ-1 Tab Control")) -> ()
        n206 = Replace Array Subset(array=w363, new element=w362, index=1) -> (w361:bool[])
      }
      frame "Akim Testi" {
        n207 = control-ref of="GKÇ-1 Akım Sonuç Tablosu"() -> (w377:refnum<vi>)
        n208 = call "Akım_Tablo_Doldur.vi"("Table Reference in"=w377, "appended array in"=w376) -> ("Test Result"=w371:bool, "Table Values"=→"GKÇ-1 Akım Sonuç Tablosu":string[][], "appended array Out"=w375:dbl[][])  [unwired: 7 in]
        n209 = local write "GKÇ-1 Tab Control"(T2."AC AKIM" ("GKÇ-1 Tab Control")) -> ()
        n210 = Replace Array Subset(array=w372, new element=w371, index=2) -> (w370:bool[])
      }
      frame "Aktif Guc Testi" {
        n211 = local write "GKÇ-1 Tab Control"(T2."AKTİF GÜÇ" ("GKÇ-1 Tab Control")) -> ()
        n212 = control-ref of="GKÇ-1 Aktif Güç Sonuç Tablosu"() -> (w385:refnum<vi>)
        n213 = call "Güç_Tablo_Doldur.vi"("Table Reference in"=w385, "Array In"=w384) -> ("Test Result"=w380:bool, "Table Values"=→"GKÇ-1 Aktif Güç Sonuç Tablosu":string[][], "Array Out"=w383:dbl[][])  [unwired: 7 in]
        n214 = Replace Array Subset(array=w381, new element=w380, index=3) -> (w379:bool[])
      }
      frame "Reaktif Guc Testi" {
        n215 = control-ref of="GKÇ-1 Reaktif Güç Sonuç Tablosu"() -> (w394:refnum<vi>)
        n216 = call "Güç_Tablo_Doldur.vi"("Table Reference in"=w394, "Array In"=w393) -> ("Test Result"=w389:bool, "Table Values"=→"GKÇ-1 Reaktif Güç Sonuç Tablosu":string[][], "Array Out"=w392:dbl[][])  [unwired: 7 in]
        n217 = Replace Array Subset(array=w390, new element=w389, index=4) -> (w388:bool[])
        n218 = local write "GKÇ-1 Tab Control"(T2."REAKTİF GÜÇ" ("GKÇ-1 Tab Control")) -> ()
      }
      frame "AC Akim Harmonik Testi" {
        n219 = control-ref of="GKÇ-1 Harmonik Akım Sonuç Tablosu"() -> (w401:refnum<vi>)
        n220 = local write "GKÇ-1 Tab Control"(T2."HARMONİK AKIM" ("GKÇ-1 Tab Control")) -> ()
        n221 = call "Harmonik_Tablo_Doldur.vi"("Table Reference in"=w401) -> ("Test Result"=w399:bool, "Table Values"=→"GKÇ-1 Harmonik Akım Sonuç Tablosu":string[][])  [unwired: 9 in]
        n222 = Replace Array Subset(array=w400, new element=w399, index=5) -> (w397:bool[])
      }
      frame "AC Gerilim Harmonik Testi" {
        n223 = local write "GKÇ-1 Tab Control"(T2."AC GERİLİM" ("GKÇ-1 Tab Control")) -> ()
        n224 = control-ref of="GKÇ-1 Harmonik Gerilim Sonuç Tablosu"() -> (w409:refnum<vi>)
        n225 = call "Harmonikgerilim_Tablo_Doldur.vi"("Table Reference in"=w409) -> ("Test Result"=w406:bool, "Table Values"=→"GKÇ-1 Harmonik Gerilim Sonuç Tablosu":string[][])  [unwired: 9 in]
        n226 = Replace Array Subset(array=w407, new element=w406, index=6) -> (w405:bool[])
      }
      frame "Flicker Testi" {
        n227 = control-ref of="GKÇ-1 Flicker Sonuç Tablosu"() -> (w420:refnum<vi>)
        n228 = call "Flicker_Tablo_Doldur.vi"("Table Reference in"=w420, "Array In"=w418) -> ("Test Result"=w414:bool, "Table Values"=→"GKÇ-1 Flicker Sonuç Tablosu":string[][], "Array Out"=w417:dbl[][])  [unwired: 7 in]
        n229 = local write "GKÇ-1 Tab Control"(T2."FLICKER" ("GKÇ-1 Tab Control")) -> ()
        n230 = Replace Array Subset(array=w415, new element=w414, index=7) -> (w413:bool[])
      }
      frame "Rapor Cikarma" {
      }
      frame "Durdur" {
      }
      frame "Ön Yükleme" {
        n231 = Index Array(array=w427) -> (element #1=→"Frekans Sonuç":bool, element #2=→"Gerilim Sonuç":bool, element #3=→"Akım Sonuç":bool, element #4=→"Aktif G. Sonuç":bool, element #5=→"Reaktif G. Sonuç":bool, element #6=→"Harmonik A. Sonuç":bool, element #7=→"Harmonik G. Sonuç":bool, element #8=→"Flicker Sonuç":bool)  [unwired: 8 in]
      }
    }
  }
  n232 = while "GKÇ-2 Display Loop" {
    tunnel: w11 -> [w440]
    tunnel: w10 -> [w439]
    stop <- w438 stop-if-true
    n233 = Wait on Notification(notifier=w440, error in (no error)=w439) -> (notification=w437:T1)  [unwired: 2 in, 3 out]
    n234 = case shown="\"Kalibratöre Baglan\"" w437 {
      tunnel: [_ _ _ _ _ _ TRUE _ _ _ _ _ _ _ _ _] -> w438
      frame "Ön Yükleme" {
      }
      frame "TSE Baslat" {
      }
      frame "Kalibratöre Baglan" {
      }
      frame "Kalibratörü Baslat" {
      }
      frame "Ön Yükleme Tamam" {
      }
      frame "Frekans Testi" {
      }
      frame "Durdur" {
      }
      frame "Gerilim Testi" {
      }
      frame "Akim Testi" {
      }
      frame "Aktif Guc Testi" {
      }
      frame "Reaktif Guc Testi" {
      }
      frame "AC Akim Harmonik Testi" {
        (unwired) Program_States."Bekleme" ("Ring")
      }
      frame "AC Gerilim Harmonik Testi" {
      }
      frame "Flicker Testi" {
      }
      frame "Rapor Cikarma" {
        (unwired) Program_States."Bekleme" ("Ring")
      }
      frame "Bekleme", Default {
      }
    }
  }
  n235 = node-c288(w7) -> ()  [unwired: 1 out]
  n236 = property class="App"() -> ("App.Kind"=w4:T9)  [unwired: 2 in, 2 out]
  n237 = case shown="\"Run Time System\"" w4 {
    tunnel: w5 -> [_ w442 w444 _ _ _ _]
    frame "invalid app kind", Default {
    }
    frame "Development System" {
      n238 = disable-structure shown="Enabled" {
        disable-tunnel: w442 -> [w443 _]
        frame Disabled {
          n239 = invoke class="VI" method="FP.Close"(reference=w443) -> ()  [unwired: 2 in, 3 out]
        }
        frame Enabled {
        }
      }
    }
    frame "Run Time System" {
      n240 = invoke class="VI" method="FP.Close"(reference=w444) -> ()  [unwired: 2 in, 3 out]
    }
    frame "Student Edition" {
    }
    frame "Embedded LabVIEW" {
    }
    frame "Evaluation" {
    }
    frame "Custom" {
    }
  }
